vi "ExposeGetData.vi"(11 "ExposeID":string) -> (2 "isnew?":bool, 3 "ExposeDataType":T1)   [LabVIEW 2017]
uses:
  ExposeDataType.ctl
  ExposeGlobals.vi
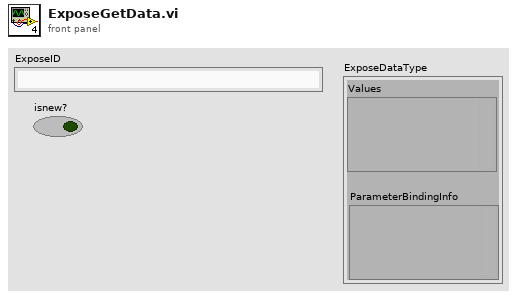
[diagram p1: front panel]
types:
  T1 = typedef "ExposeDataType.ctl" = cluster{"Values":variant, "ParameterBindingInfo":variant}
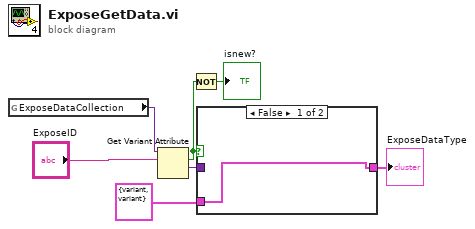
[diagram p0: block diagram]
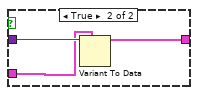
[diagram p2: hidden frame]
diagram:
  n1 = global read "ExposeGlobals.vi" "ExposeDataCollection"() -> (w6:variant)
  n2 = Get Variant Attribute(Variant=w6, name="ExposeID") -> (found=w4:bool, value=w3:variant)  [unwired: 2 in, 2 out]
  n3 = Not(x=w4) -> (.not. x?=→"isnew?":bool)
  n4 = case shown="False" w4 {
    tunnel: w3 -> [_ w11]
    tunnel: T1 {"Values"=variant, "ParameterBindingInfo"=variant} ("ExposeDataType") -> [w8 w10]
    tunnel: [w8 w9] -> w1
    frame False {
    }
    frame True {
      n5 = Variant To Data(type=w10, Variant=w11) -> (data=w9:T1)  [unwired: 1 in, 1 out]
    }
  }
  "ExposeDataType" <- w1
